vi "delete function from configuration.vi"(8 "error in":errorcluster, 10 "index":i32, 11 "tag bus configurable plugin module configuration in":refnum<class "tag bus processing plugin module configuration.lvclass">) -> (0 "error out":errorcluster, 2 "function deleted":T1, 3 "tag bus configurable plugin module configuration out":refnum<class "tag bus processing plugin module configuration.lvclass">)   [LabVIEW 2013, in "tag bus processing plugin module configuration.lvclass"]
uses:
  tag bus processing plugin module configuration.lvclass
  processing channels.ctl
  <vilib>/NI/Tag Bus Module Framework/channel/TBM channel.lvclass
  tag bus processing plugin module configuration.lvclass/tag bus processing plugin module configuration.ctl
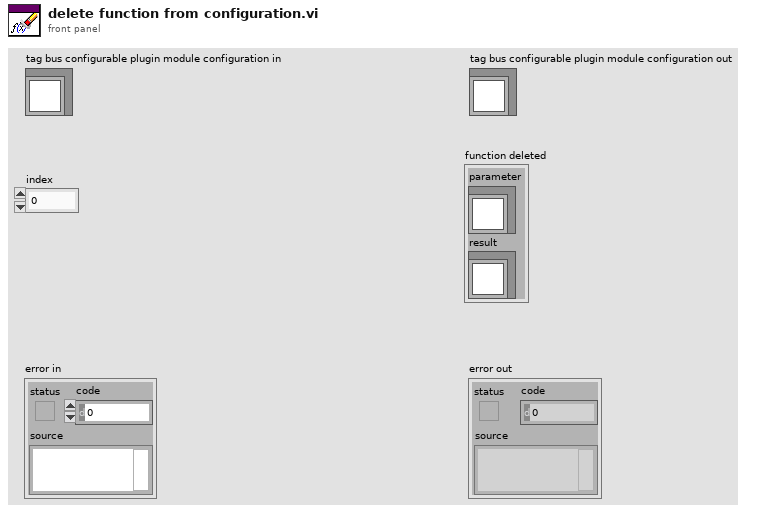
[diagram p1: front panel]
types:
  T1 = typedef "tag bus processing plugin module configuration.lvclass/processing channels.ctl" = cluster{"parameter":refnum<class "TBM channel.lvclass">, "result":refnum<class "TBM channel.lvclass">}
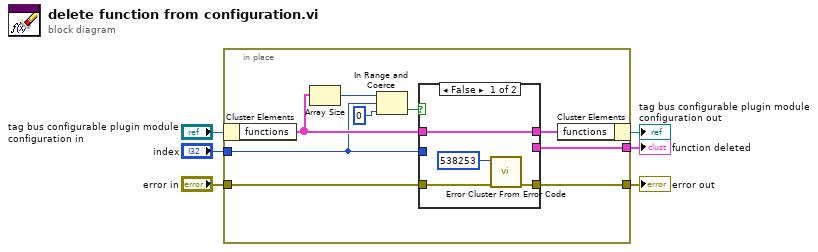
[diagram p0: block diagram]
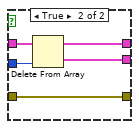
[diagram p2: hidden frame]
diagram:
  n1 = in-place {
    in-place-border: "index" -> [w8]
    in-place-border: [w10] -> w3
    in-place-border: "error in" -> [w9]
    in-place-border: [w7] -> w1
    n2 = in-place-cluster #1("tag bus configurable plugin module configuration in") -> ("functions"=w11:T1[])
    n3 = Array Size(array=w11) -> (size(s)=w15:i32)
    n4 = In Range and Coerce(upper limit=w15, x=w8, lower limit=0) -> (In Range?=w13:bool)  [unwired: 1 out]
    n5 = case shown="False" w13 {
      tunnel: [w19 w22] -> w12
      tunnel: w11 -> [w19 w23]
      tunnel: [w18 w24] -> w10
      tunnel: w9 -> [w17 w24]
      tunnel: w8 -> [_ w21]
      tunnel: [_ w20] -> w7
      frame False {
        n6 = call <vilib>:"Error Cluster From Error Code.vi"("error in (no error)"=w17, "error code (0)"=538253) -> ("error out"=w18:errorcluster)  [unwired: 7 in]
      }
      frame True {
        n7 = Delete From Array(array=w23, index=w21) -> (deleted portion=w20:T1, array with subset deleted=w22:T1[])  [unwired: 1 in]
      }
    }
    n8 = in-place-cluster #1("functions"=w12) -> (→"tag bus configurable plugin module configuration out":refnum<class "tag bus processing plugin module configuration.lvclass">)
  }
  "error out" <- w3
  "function deleted" <- w1
